vi "ARM_ACT.vi"(8 "error in":errorcluster) -> (0 "error out":errorcluster)   [LabVIEW 2023]
uses:
  <vilib>/Rock Robotics/WPI/ThirdParty/Phoenix-LabVIEW/Motor Controller/Controls/CTRE_Phoenix_MotorControl_ControlMode.ctl
  <vilib>/Rock Robotics/Network Tables/NT Read Number.vi
  <vilib>/Rock Robotics/Network Tables/NT Read Boolean.vi
  ARM_GLOBALS.vi
  <vilib>/Rock Robotics/Network Tables/NT Read Numeric Array.vi
  <vilib>/Rock Robotics/Network Tables/NT Write Number.vi
  <vilib>/Rock Robotics/WPI/ThirdParty/JAS_Junk/TrajLib/Trajectory_Library.lvlib
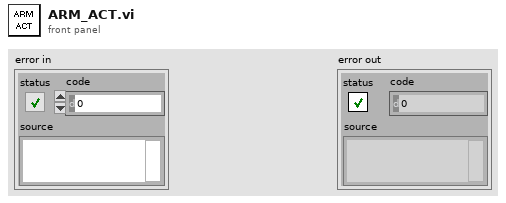
[diagram p1: front panel]
types:
  T1 = cluster{"Kg_Gravity_gain":dbl, "phi_Equilibrium_phase_Deg":dbl, "Ks":dbl}
  T2 = typedef "CTRE_Phoenix_MotorControl_ControlMode.ctl" = u16
  T3 = typedef "Trajectory_Library.lvlib/DCMOTOR_TYPES_ENUM.ctl" = enum16{"CIM", "AndyMark 9015", "Andy Mark RS 775 125", "Bag", "BaneBots RS 550", "BaneBots RS 775", "Falcon 500", "Mini CIM", "NEO", "NEO 550", "Romi BuiltIn", "Vex 775 Pro", "Snow Blower AM 2235A", "Bosch Seat AM 3493"}
  T4 = cluster{"Numeric":dbl, "Numeric":dbl, "Numeric":dbl}
  T5 = typedef "Trajectory_Library.lvlib/LINEAR_SYSTEM_ID_SINGLE_JOINT_ARM_MODEL.ctl" = cluster{"DCMOTOR_TYPES":T3, "Num Motors":i32, "ArmLength_M":dbl, "massKg":dbl, "Gearing":dbl, "MOI kgm2":dbl, "Estimate MOI":bool}
  T6 = typedef "Trajectory_Library.lvlib/LINEAR_SYSTEM_LOOP_SNGJNTARM_CTRL_PARAMS.ctl" = cluster{"Ang Model Std Dev Rad":dbl, "Ang Meas Std Dev Rad":dbl, "Ang Ctrl Tol Rad":dbl, "Max Ctrl Out V":dbl, "Vel Model Std Dev Rad/Sec":dbl, "Vel Ctrl Tol Rad/Sec":dbl}
  T7 = typedef "WPI_MotorControlDeviceRef.ctl" = cluster{"DeviceStatus":errorcluster, "Type":T8, "PWM":cluster{"PWM Channel":T9, "DeadBand":T10}, "CAN":cluster{"Device Number":u8, "SetOutput VI Ref":variant, "GetOutput VI Ref":variant, "Enable VI Ref":variant, "Disable VI Ref":variant, "Data":variant}, "Invert":bool, "DIO PWM":cluster{"PWM \"Enable\" Channel":T9, "DIOChannel":T11, "PWM Rate":dbl}}
  T8 = typedef "WPI_MotorControlType.ctl" = enum16{"PWM", "CAN", "DIO PWM"}
  T9 = typedef "FPGA_DIOPWMChannel.ctl" = enum8{"PWM 0", "PWM 1", "PWM 2", "PWM 3", "PWM 4", "PWM 5", "PWM 6", "PWM 7", "PWM 8", "PWM 9", "PWM MXP 0", "PWM MXP 1", "PWM MXP 2", "PWM MXP 3", "PWM MXP 4", "PWM MXP 5", "PWM MXP 6", "PWM MXP 7", "PWM MXP 8", "PWM MXP 9", "Invalid"}
  T10 = typedef "WPI_PWMDeadband.ctl" = cluster{"Name":string, "maxPositivePwm":i32, "minPositivePwm":i32, "centerPwm":i32, "maxNegativePwm":i32, "minNegativePwm":i32, "angularRange":u16}
  T11 = typedef "FPGA_DIOChannel.ctl" = enum8{"DIO 0", "DIO 1", "DIO 2", "DIO 3", "DIO 4", "DIO 5", "DIO 6", "DIO 7", "DIO 8", "DIO 9", "DIO MXP 0", "DIO MXP 1", "DIO MXP 2", "DIO MXP 3", "DIO MXP 4", "DIO MXP 5", "DIO MXP 6", "DIO MXP 7", "DIO MXP 8", "DIO MXP 9", "DIO MXP 10", "DIO MXP 11", "DIO MXP 12", "DIO MXP 13", "DIO MXP 14", "DIO MXP 15", "SPI Port CS1", "SPI Port CS2", "SPI Port CS3", "SPI Port MISO", "SPI Port MOSI", "Invalid"}
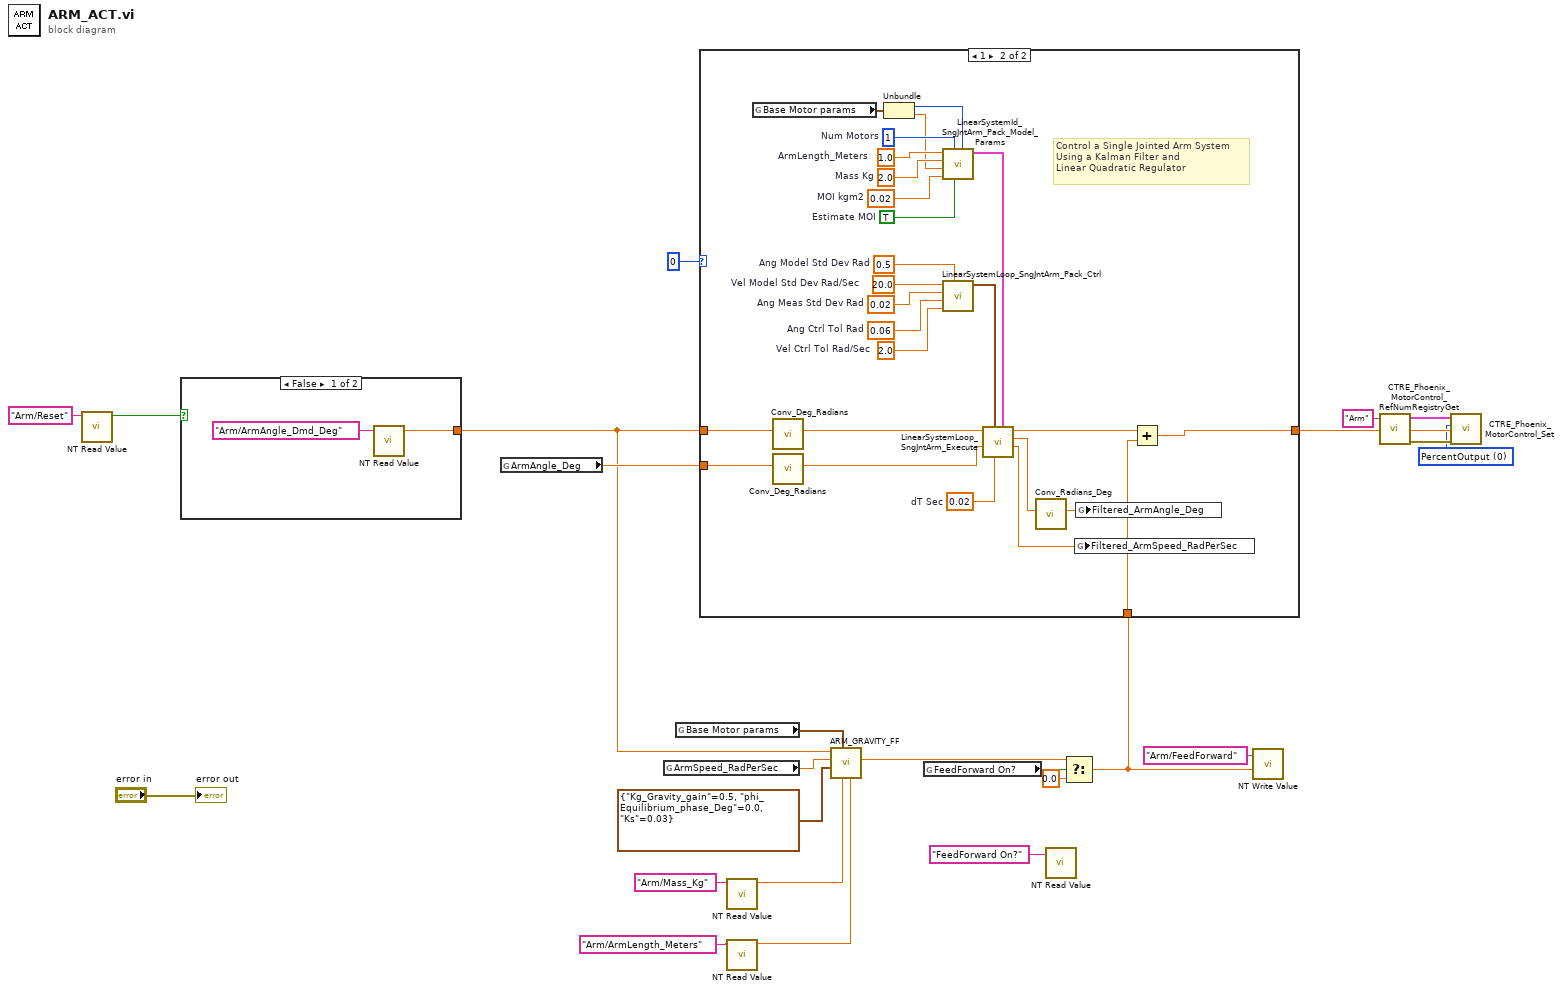
[diagram p0: block diagram]
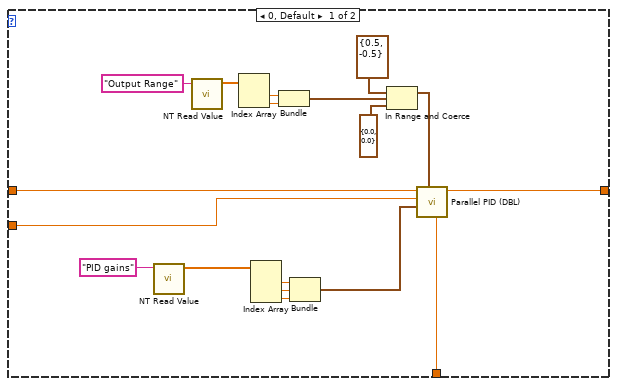
[diagram p2: hidden frame]
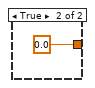
[diagram p3: hidden frame]
diagram:
  w3 = T2 0 items=["PercentOutput"=0, "Position"=1, "Velocity"=2, "Current"=3, "Follower"=5, "MotionProfile"=6, "MotionMagic"=7, "MotionProfileArc"=10, "Disabled"=15] ("Control Mode")
  n1 = call-poly <vilib>:"NT Read Value.vi"("name"="Arm/Reset") -> ("value"=w23:bool)  [unwired: 8 in, 2 out]
  n2 = case shown="False" w23 {
    tunnel: [w26 0.0 ("value")] -> w12
    frame False {
      n3 = call-poly <vilib>:"NT Read Value.vi"("name"="Arm/ArmAngle_Dmd_Deg") -> ("value"=w26:dbl)  [unwired: 8 in, 2 out]
    }
    frame True {
    }
  }
  n4 = global read "ARM_GLOBALS.vi" "ArmAngle_Deg"() -> (w14:dbl)
  n5 = global read "ARM_GLOBALS.vi" "ArmSpeed_RadPerSec"() -> (w9:dbl)
  n6 = global read "ARM_GLOBALS.vi" "Base Motor params"() -> (w5:cluster{"Motor Type":T3, "Gear Ratio":dbl})
  n7 = call-poly <vilib>:"NT Read Value.vi"("name"="Arm/Mass_Kg") -> ("value"=w7:dbl)  [unwired: 8 in, 2 out]
  n8 = call-poly <vilib>:"NT Read Value.vi"("name"="Arm/ArmLength_Meters") -> ("value"=w6:dbl)  [unwired: 8 in, 2 out]
  n9 = call "ARM_GRAVITY_FF.vi"("ArmLength_M"=w6, "Mass_Kg"=w7, "Motor Params"=w5, "FF params"=T1 {"Kg_Gravity_gain"=0.5, "phi_Equilibrium_phase_Deg"=0.0, "Ks"=0.03}, "ArmSpeed_Dmd_RadPerSec"=w9, "ArmAngle_Dmd_Deg"=w12) -> ("FeedForward"=w10:dbl)  [unwired: 5 in]
  n10 = global read "ARM_GLOBALS.vi" "FeedForward On?"() -> (w13:bool)
  n11 = call-poly <vilib>:"NT Read Value.vi"("name"="FeedForward On?") -> ()  [unwired: 8 in, 3 out]
  n12 = Select(t=w10, s=w13, f=0.0) -> (s? t:f=w11:dbl)
  n13 = case shown="1" 0 {
    tunnel: w14 -> [w37 w58]
    tunnel: w12 -> [w36 w59]
    tunnel: w11 -> [w35 w54]
    tunnel: [w34 w55] -> w4
    frame 0, Default {
      n14 = call-poly <vilib>:"NT Read Value.vi"("name"="PID gains") -> ("value"=w32:dbl[])  [unwired: 8 in, 2 out]
      n15 = call-poly <vilib>:"NT Read Value.vi"("name"="Output Range") -> ("value"=w39:dbl[])  [unwired: 8 in, 2 out]
      n16 = Index Array(array=w39) -> (element #1=w40:dbl, element #2=w41:dbl)  [unwired: 2 in]
      n17 = Index Array(array=w32) -> (element #1=w31:dbl, element #2=w30:dbl, element #3=w29:dbl)  [unwired: 3 in]
      n18 = Bundle("Numeric"=w40, "Numeric"=w41) -> (w42:cluster{"Numeric":dbl, "Numeric":dbl})  [unwired: 1 in]
      n19 = Bundle("Numeric"=w31, "Numeric"=w30, "Numeric"=w29) -> (w28:T4)  [unwired: 1 in]
      n20 = In Range and Coerce(upper limit=cluster{"Numeric":dbl, "Numeric":dbl} {"Numeric"=0.5, "Numeric"=-0.5}, x=w42, lower limit=cluster{"Numeric":dbl, "Numeric":dbl} {"Numeric"=0.0, "Numeric"=0.0}) -> (coerced(x)=w45:cluster{"Numeric":dbl, "Numeric":dbl})  [unwired: 1 out]
      n21 = call <vilib>:"Parallel PID (DBL).vi"("FeedFwd Value"=w35, "output range"=w45, "PID gains"=w28, "process variable"=w37, "setpoint"=w36) -> ("output"=w34:dbl)  [unwired: 3 in, 3 out]
    }
    frame 1 {
      w52 = 0.02  # dT Sec
      w61 = 20.0  # Vel Model Std Dev Rad/Sec
      w60 = 0.02  # Ang Meas Std Dev Rad
      w62 = 0.06  # Ang Ctrl Tol Rad
      w63 = 2.0  # Vel Ctrl Tol Rad/Sec
      w64 = 0.5  # Ang Model Std Dev Rad
      w67 = TRUE  # Estimate MOI
      w68 = 0.02  # MOI kgm2
      w69 = 1.0  # ArmLength_Meters
      w70 = 2.0  # Mass Kg
      w71 = 1  # Num Motors
      # "Control a Single Jointed Arm System\nUsing a Kalman Filter and \nLinear Quadratic Regulator"
      n22 = global read "ARM_GLOBALS.vi" "Base Motor params"() -> (w51:cluster{"Motor Type":T3, "Gear Ratio":dbl})
      n23 = call <vilib>:"Conv_Deg_Radians.vi"("Degress"=w59) -> ("Radians"=w57:dbl)  [unwired: 10 in]
      n24 = call <vilib>:"Conv_Deg_Radians.vi"("Degress"=w58) -> ("Radians"=w56:dbl)  [unwired: 10 in]
      n25 = Unbundle(w51) -> ("Motor Type"=w50:T3, "Gear Ratio"=w49:dbl)
      n26 = call <vilib>:"LinearSystemId_SngJntArm_Pack_Model_Params.vi"("DCMOTOR_TYPES"=w50, "Estimate MOI"=w67, "Num Motors"=w71, "MOI kgm2"=w68, "Gearing"=w49, "massKg"=w70, "ArmLength_M"=w69) -> ("SngJntArmSim_Model _Params"=w66:T5)  [unwired: 4 in]
      n27 = call <vilib>:"LinearSystemLoop_SngJntArm_Pack_Ctrl.vi"("Ang Model Std Dev Rad"=w64, "Vel Ctrl Tol Rad/Sec"=w63, "Ang Ctrl Tol Rad"=w62, "Ang Meas Std Dev Rad"=w60, "Vel Model Std Dev Rad/Sec"=w61) -> ("LinearSystemLoop_SngJntArm_Ctrl_Params"=w65:T6)  [unwired: 6 in]
      n28 = call <vilib>:"LinearSystemLoop_SngJntArm_Execute.vi"("LinearSystem_ID_SngJntArm_Model"=w66, "dT Sec"=w52, "LinearSystem_SngJntArm_Ctrl_Params"=w65, "Process Variable\nRadians"=w56, "Ang Pos SP Rad"=w57) -> ("Filtered Vel Rad/Sec"=w46:dbl, "Filtered Angle Radians"=w48:dbl, "Motor Dmd"=w53:dbl)  [unwired: 2 in, 2 out]
      n29 = call <vilib>:"Conv_Radians_Deg.vi"("Radians"=w48) -> ("Degrees"=w47:dbl)  [unwired: 10 in]
      n30 = global write "ARM_GLOBALS.vi" "Filtered_ArmSpeed_RadPerSec"(w46) -> ()
      n31 = global write "ARM_GLOBALS.vi" "Filtered_ArmAngle_Deg"(w47) -> ()
      n32 = Add(x=w53, y=w54) -> (x+y=w55:dbl)
    }
  }
  n33 = call-poly <vilib>:"NT Write Value.vi"("value"=w11, "name"="Arm/FeedForward") -> ()  [unwired: 9 in, 1 out]
  n34 = call <vilib>:"CTRE_Phoenix_MotorControl_RefNumRegistryGet.vi"("refnum name"="Arm") -> ("error out"=w18:errorcluster, "PhoenixMotorControlDevRef"=w19:T7)  [unwired: 9 in]
  n35 = call <vilib>:"CTRE_Phoenix_MotorControl_Set.vi"("error in (no error)"=w18, "Output"=w4, "Control Mode"=w3, "PhoenixMotorControlDevRef"=w19) -> ()  [unwired: 6 in, 2 out]
  "error out" <- "error in"
